vi "SSL_get_peer_certificate.vi"(8 "error in (no error)":errorcluster, 11 "SSL-Lib in":refnum<class "SSL.lvclass">) -> (0 "error out":errorcluster, 2 "X509-Cert out":refnum<class "X509-Cert.lvclass">, 3 "SSL-Lib out":refnum<class "SSL.lvclass">)   [LabVIEW 2013, in "SSL_Lib.lvlib" / "SSL.lvclass"]
uses:
  SSL.lvclass
  X509-Cert/X509-Cert.lvclass
  SSL-Lib/SSL-Lib.lvclass/SSL-Lib.ctl
  SSL.lvclass/SSL.ctl
  X509-Cert/X509-Cert.lvclass/X509-Cert.ctl
  X509-Cert/Write Handle.vi
  SSL-Lib/Read SSL Library Path.vi
  Read Handle.vi
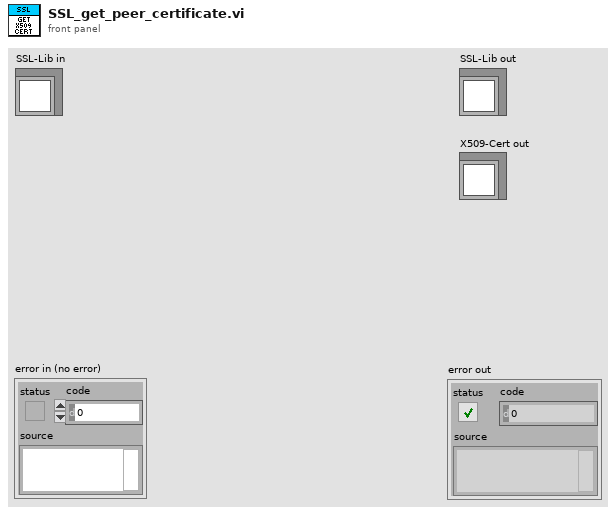
[diagram p1: front panel]
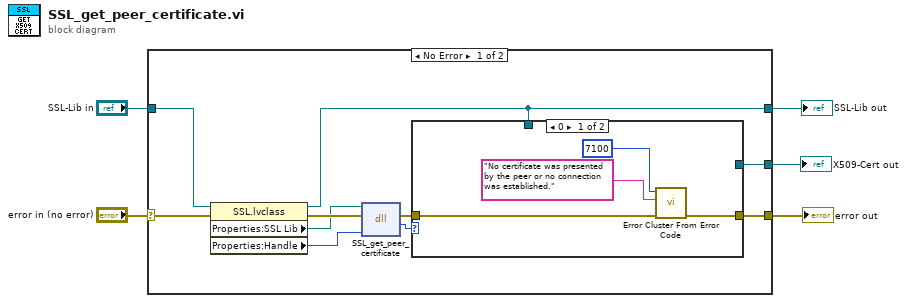
[diagram p0: block diagram]
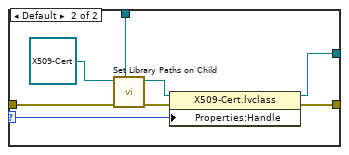
[diagram p2: hidden frame]
diagram:
  n1 = case shown="No Error" "error in (no error)" {
    selector: "error in (no error)" -> [w15 w28]
    tunnel: [w7 w29] -> w3
    tunnel: "SSL-Lib in" -> [w11 w29]
    tunnel: [w8 w28] -> w2
    tunnel: [w6 _] -> w1
    frame No Error {
      n2 = property class="SSL.lvclass"(reference=w11, error in=w15) -> (reference out=w7:refnum<class "SSL.lvclass">, error out=w14:errorcluster, "Properties:SSL Lib"=w13:path, "Properties:Handle"=w12:u64)
      n3 = dll-call lib="C:/Program Files (x86)/National Instruments/Shared/nissl/NIssleay32.dll" fn="SSL_get_peer_certificate"(path in=w13, error in=w14, "SSL"=w12) -> (error out=w9:errorcluster, "return type"=w10:u64)  [unwired: 2 in, 1 out]
      n4 = case shown="0" w10 {
        selector: w10 -> [_ w21]
        tunnel: w9 -> [w19 w24]
        tunnel: [w18 w27] -> w8
        tunnel: w7 -> [_ w22]
        tunnel: [_ w20] -> w6
        frame 0 {
          n5 = call <vilib>:"Error Cluster From Error Code.vi"("error in (no error)"=w19, "error message (\"\")"="No certificate was presented by the peer or no connection was established." ("error message (\"\")"), "error code (0)"=7100) -> ("error out"=w18:errorcluster)  [unwired: 6 in]
        }
        frame Default {
          n6 = call-dynamic "Set Library Paths on Child.vi"(7:"SSL-Lib in"=w22, "error in (no error)"=w24, 11:"SSL-Lib in"=refnum<class "X509-Cert.lvclass"> refnum ("SSL_Lib.lvlib:X509-Cert.lvclass")) -> ("error out"=w23:errorcluster, "SSL-Lib out"=w26:refnum<class "X509-Cert.lvclass">)  [unwired: 7 in]
          n7 = property class="X509-Cert.lvclass"(reference=w26, error in=w23, "Properties:Handle"=w21) -> (reference out=w20:refnum<class "X509-Cert.lvclass">, error out=w27:errorcluster)
        }
      }
    }
    frame Error {
    }
  }
  "SSL-Lib out" <- w3
  "error out" <- w2
  "X509-Cert out" <- w1
